vi "Leap Motion - Spread shape data.vi"(8 "Error In":errorcluster, 10 "Spread  Button 2":bool) -> (0 "Error Out":errorcluster, 2 "Spread":u8)   [LabVIEW 2014]
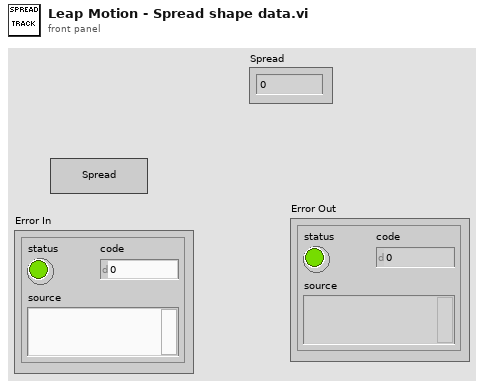
[diagram p1: front panel]
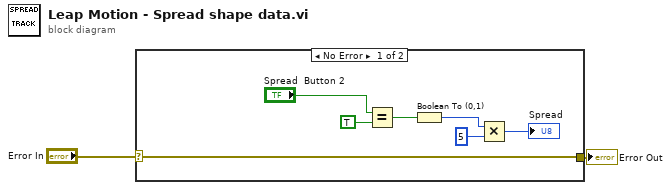
[diagram p0: block diagram]
diagram:
  n1 = case shown="No Error" "Error In" {
    selector: "Error In" -> [w9 w10]
    tunnel: [w9 w10] -> w1
    frame No Error {
      n2 = Equal?(x="Spread  Button 2", y=TRUE) -> (x = y?=w6:bool)
      n3 = Boolean To (0,1)(Boolean=w6) -> (0, 1=w5:i16)
      n4 = Multiply(x=w5, y=i16 5) -> (x*y=→"Spread":i16)
    }
    frame Error {
    }
  }
  "Error Out" <- w1
